vi "Pad 1d array with wrap around data (dbl).vi"(9 "Pad Points":i32, 11 "Array":dbl[](array[numeric])) -> (1 "Pad Size":i32, 2 "Original Size":i32, 3 "Padded Array":dbl[](array[numeric]))   [LabVIEW 2010]
doc: "Wraps data by specified percent"
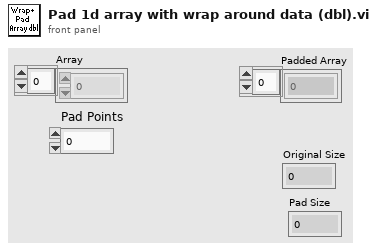
[diagram p1: front panel]
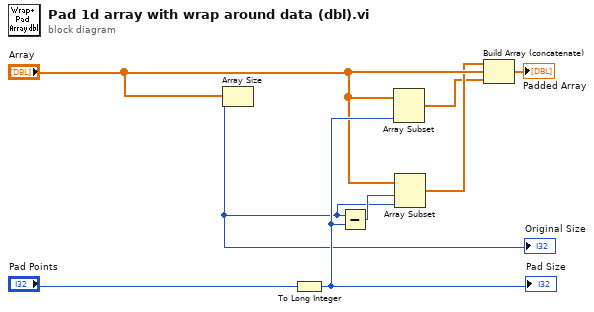
[diagram p0: block diagram]
diagram:
  n1 = Array Size(array="Array") -> (size(s)=w2:i32)
  "Original Size" <- w2
  n2 = To Long Integer(number="Pad Points") -> (32bit integer=w8:i32)
  "Pad Size" <- w8
  n3 = Subtract(x=w2, y=w8) -> (x-y=w3:i32)
  n4 = Array Subset(array="Array", length=w8) -> (w4:dbl[])  [unwired: 1 in]
  n5 = Array Subset(array="Array", index=w3, length=w2) -> (w5:dbl[])
  n6 = Build Array (concatenate)(w5, "Array", w4) -> (→"Padded Array":dbl[])
